vi "Fetch Multi Eval Meas List Power Monitor Results Segment Location.vi"(8 "error in (no error)":errorcluster, 9 "Segment (1)":T1=1, 10 "Instance (1)":T2=1, 11 "VISA resource name":refnum<visa-resource-name>) -> (0 "error out":errorcluster, 1 "Segment Start":i32, 2 "Reliability":i32, 3 "VISA resource name out":refnum<visa-resource-name>, 4 "Segment Length":i32)   [LabVIEW 2020, in "Rohde&Schwarz CMWXP NR FR1 Measurement.lvlib"]
doc: "Returns the location of the power monitor results for segment <no> within a result list for all measured segments. Such a result list is, for example, returned by rscmwxpnrfr1m Fetch Multi Eval Meas List Power Monitor RMS Results.vi and rscmwxpnrfr1m Fetch Multi Eval Meas List Power Monitor Peak Results.vi.\n\nAttributes:\nRSCMWXPNRFR1M_ATTR_FETCH_MULTI_EVAL_MEAS_LIST_POWER_MONITOR_RESULTS_SEGMENT_START\nRSCMWXPNRFR1M_ATTR_FETCH_MULTI_EVAL_MEAS_LIST_POWER_MONITOR_RESULTS_SEGMENT_LENGTH\n\nRemote-control commands:\nFETCh:NRSub:MEAS<i>:MEValuation:LIST:SEGMent<no>:PMONitor:ARRay:STARt?\nFETCh:NRSub:MEAS<i>:MEValuation:LIST:SEGMent<no>:PMONitor:ARRay:LENGth?"
uses:
  <instrlib>/Rohde&Schwarz CMWXP NR FR1 Measurement/Rohde&Schwarz CMWXP NR FR1 Measurement.lvlib
  <instrlib>/Rohde&Schwarz CMWXP NR FR1 Measurement/Private/_Instance.ctl
  <instrlib>/Rohde&Schwarz CMWXP NR FR1 Measurement/Private/_Segment.ctl
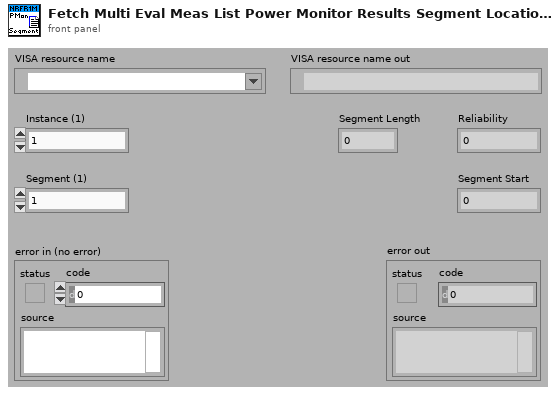
[diagram p1: front panel]
types:
  T1 = typedef "Rohde&Schwarz CMWXP NR FR1 Measurement.lvlib/_Segment.ctl" = i32
  T2 = typedef "Rohde&Schwarz CMWXP NR FR1 Measurement.lvlib/_Instance.ctl" = i32
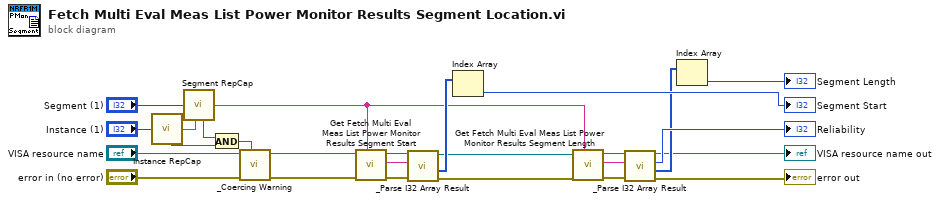
[diagram p0: block diagram]
diagram:
  n1 = call <instrlib>:"Instance RepCap.vi"("Instance In"="Instance (1)") -> ("In Range?"=w22:bool, "RepCap Identifier Out"=w21:string)  [unwired: 1 in]
  n2 = call <instrlib>:"Segment RepCap.vi"("Segment In"="Segment (1)", "RepCap String In (\"\")"=w21) -> ("In Range?"=w20:bool, "RepCap Identifier Out"=w10:string)
  n3 = And(x=w20, y=w22) -> (x .and. y?=w24:bool)
  n4 = call <instrlib>:"_Coercing Warning.vi"("In Range?"=w24, "error in (no error)"="error in (no error)", "VISA resource name"="VISA resource name") -> ("error out"=w18:errorcluster, "VISA resource name out"=w19:refnum<visa-resource-name>)  [unwired: 7 in]
  n5 = call "Get Fetch Multi Eval Meas List Power Monitor Results Segment Start"("Repeated Capabilities"=w10, "error in (no error)"=w18, "instrument handle"=w19) -> ("error out"=w15:errorcluster, "Fetch Multi Eval Meas List Power Monitor Results Segment Start"=w16:string, "instrument handle out"=w17:refnum<visa-resource-name>)  [unwired: 6 in]
  n6 = call <instrlib>:"_Parse I32 Array Result.vi"("error in (no error)"=w15, "Input String"=w16, "VISA resource name"=w17) -> ("error out"=w11:errorcluster, "Results"=w14:i32[], "VISA resource name out"=w12:refnum<visa-resource-name>)  [unwired: 5 in, 1 out]
  n7 = Index Array(array=w14) -> (element=→"Segment Start":i32)  [unwired: 1 in]
  n8 = call "Get Fetch Multi Eval Meas List Power Monitor Results Segment Length"("Repeated Capabilities"=w10, "error in (no error)"=w11, "instrument handle"=w12) -> ("error out"=w7:errorcluster, "Fetch Multi Eval Meas List Power Monitor Results Segment Length"=w8:string, "instrument handle out"=w9:refnum<visa-resource-name>)  [unwired: 6 in]
  n9 = call <instrlib>:"_Parse I32 Array Result.vi"("error in (no error)"=w7, "Input String"=w8, "VISA resource name"=w9) -> ("error out"=→"error out":errorcluster, "Results"=w5:i32[], "Reliability"=→"Reliability":i32, "VISA resource name out"=→"VISA resource name out":refnum<visa-resource-name>)  [unwired: 5 in]
  n10 = Index Array(array=w5) -> (element=→"Segment Length":i32)  [unwired: 1 in]
